vi "fgv_cap_ctrl-ref.vi"(7 "cmd":T2, 11 "input cluster":T1) -> (3 "input cluster 2":T1)   [LabVIEW 2019]
uses:
  _ctrl/rw.ctl
  ref_cap_ctrl-ref.ctl
  cap_config.ctl
  Breakdown-Spec.ctl
panel:
  in  "Breakdown-Spec":refnum<vi>
  # "제어단"
  # "출력단"
  # "온도기준"
  # "제어단 전압"
  # "출력단 전원"
  # "DL950"
  # "Discharge"
  # "Test Cycle"
  # "작동 설정"
  # "제어단 전압"
  # "출력단 전원"
  # "DL950"
  # "Discharge"
  # "Test Cycle"
  # "작동 설정"
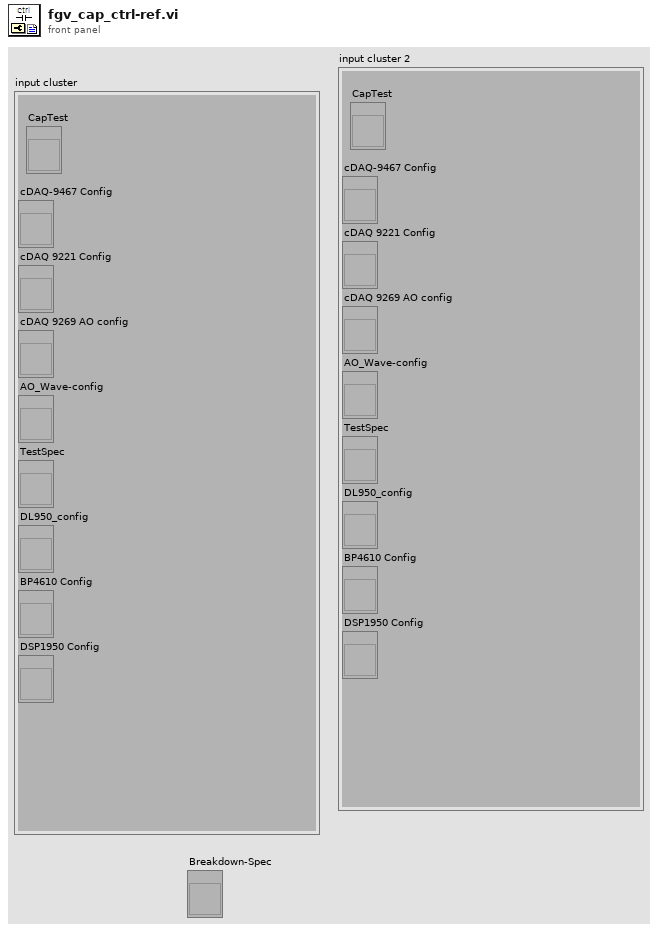
[diagram p1: front panel]
types:
  T1 = typedef "ref_cap_ctrl-ref.ctl" = cluster{"cDAQ-9467 Config":refnum<vi>, "cDAQ 9221 Config":refnum<vi>, "cDAQ 9269 AO config":refnum<vi>, "AO_Wave-config":refnum<vi>, "TestSpec":refnum<vi>, "DL950_config":refnum<vi>, "BP4610 Config":refnum<vi>, "DSP1950 Config":refnum<vi>, "CapTest":refnum<vi>}
  T2 = typedef "rw.ctl" = enum16{"read", "write"}
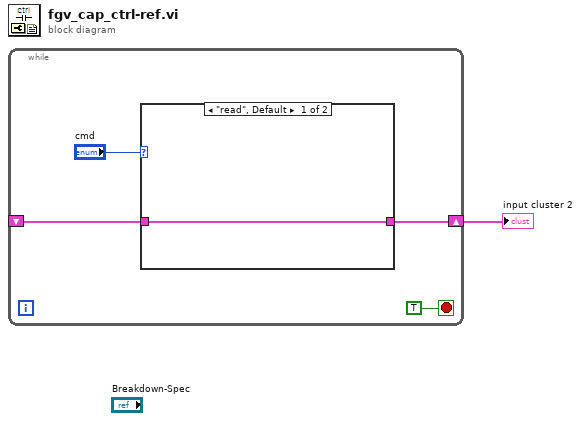
[diagram p0: block diagram]
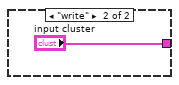
[diagram p2: hidden frame]
diagram:
  n1 = while {
    shift-right: [w3] -> w1
    shift-left: _ -> [w2]
    stop <- TRUE stop-if-true
    n2 = case shown="\"read\", Default" "cmd" {
      tunnel: [w6 "input cluster"] -> w3
      tunnel: w2 -> [w6 _]
      frame "read", Default {
      }
      frame "write" {
      }
    }
  }
  "input cluster 2" <- w1
